vi "configure_measurement.vi"() -> ()   [LabVIEW 2020]
panel:
  out "String":string
  in  "Resistance Range Upper Limit (2E+8 Ohm)":dbl=200000000.0
  in  "Resistance Range Lower Limit (2 Ohm)":dbl=2.0
  in  "Resistance Auto Range (T: Enable)":bool=TRUE
  in  "Channel (0: Channel 1)":i32(ring) items=["Channel 1", "Channel 2"]
  in  "Enable Resistance Compensation (F: Disable)":bool
  in  "Resistance Measurement Mode (1: Auto)":i32(ring)=1 items=["Manual", "Auto"]
  in  "Resistance Range (2 Ohm)":dbl=2.0
  in  "Resistance NPLC (0.1)":dbl=0.1
  in  "Auto Resistance NPLC (F: Disable)":bool
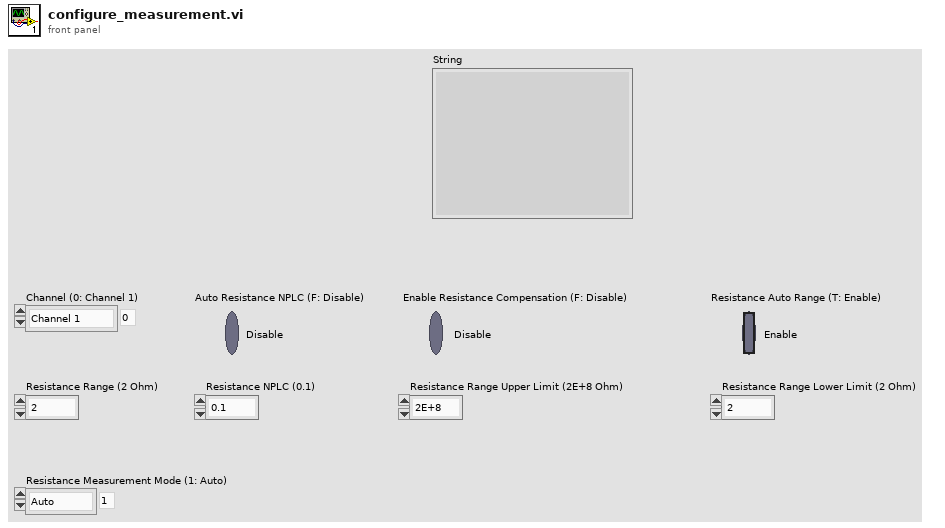
[diagram p1: front panel]
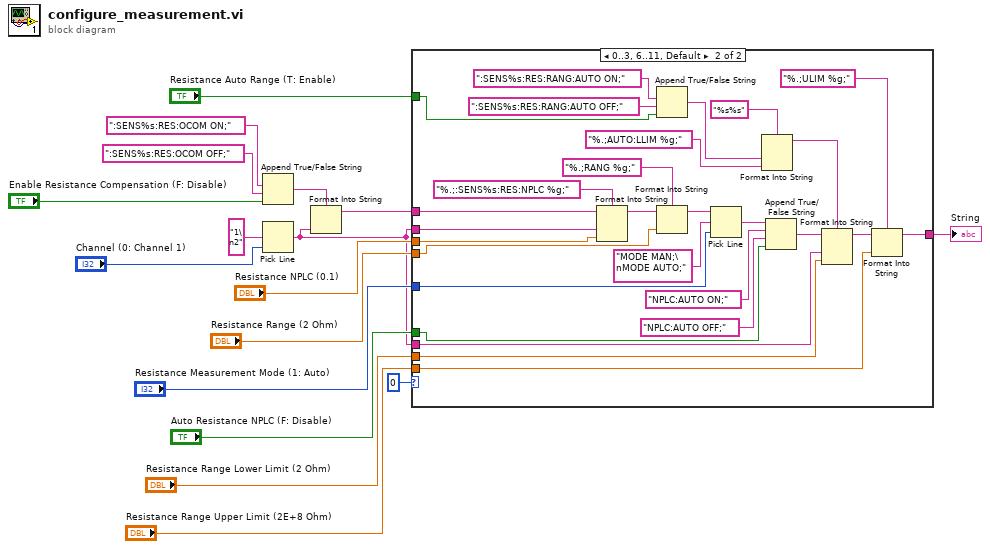
[diagram p0: block diagram]
diagram:
  n1 = Append True/False String(1:"Enable Resistance Compensation (F: Disable)", 2:":SENS%s:RES:OCOM OFF;", 3:":SENS%s:RES:OCOM ON;") -> (0:w3:string)  [unwired: 1 in]
  n2 = Pick Line(multi-line string="1\n2" ("string (\"\")"), line index="Channel (0: Channel 1)") -> (output string=w7:string)  [unwired: 1 in]
  n3 = Format Into String(format string=w3, w7) -> (resulting string=w4:string)  [unwired: 2 in, 1 out]
  n4 = case shown="0..3, 6..11, Default" u16 0 ("B2900 Series Mode") {
    tunnel: w7 -> [_ w29]
    tunnel: "Resistance Range (2 Ohm)" -> [_ w28]
    tunnel: "Resistance NPLC (0.1)" -> [_ w27]
    tunnel: "Resistance Measurement Mode (1: Auto)" -> [_ w26]
    tunnel: "Auto Resistance NPLC (F: Disable)" -> [_ w25]
    tunnel: "Resistance Auto Range (T: Enable)" -> [_ w24]
    tunnel: w7 -> [_ w23]
    tunnel: "Resistance Range Lower Limit (2 Ohm)" -> [_ w22]
    tunnel: "Resistance Range Upper Limit (2E+8 Ohm)" -> [_ w21]
    tunnel: [w18 w20] -> w1
    tunnel: w4 -> [w18 w19]
    frame 4, 5, 12, 13 {
      # "Commands in this case are\napplicable for Agilent B2961A,B2962A, B2961B, B2962B."
    }
    frame 0..3, 6..11, Default {
      n5 = Format Into String(format string="%.;:SENS%s:RES:NPLC %g;", initial string=w19, w29, w27) -> (resulting string=w33:string)  [unwired: 1 in, 1 out]
      n6 = Append True/False String(1:w24, 2:":SENS%s:RES:RANG:AUTO OFF;", 3:":SENS%s:RES:RANG:AUTO ON;") -> (0:w42:string)  [unwired: 1 in]
      n7 = Format Into String(format string="%.;RANG %g;", initial string=w33, w28) -> (resulting string=w36:string)  [unwired: 1 in, 1 out]
      n8 = Pick Line(string ("")=w36, multi-line string="MODE MAN;\nMODE AUTO;", line index=w26) -> (output string=w46:string)
      n9 = Format Into String(format string="%s%s", w42, "%.;AUTO:LLIM %g;") -> (resulting string=w44:string)  [unwired: 2 in, 1 out]
      n10 = Append True/False String(1:w25, 2:"NPLC:AUTO OFF;", 3:"NPLC:AUTO ON;", 4:w46) -> (0:w40:string)
      n11 = Format Into String(format string=w44, initial string=w40, w23, w22) -> (resulting string=w39:string)  [unwired: 1 in, 1 out]
      n12 = Format Into String(format string="%.;ULIM %g;", initial string=w39, w21) -> (resulting string=w20:string)  [unwired: 1 in, 1 out]
    }
  }
  "String" <- w1
